vi "File HDF5 Close.vi"(8 "error in (no error)":errorcluster, 11 "HDF IDs in":T1) -> (0 "error out":errorcluster)   [LabVIEW 2011]
uses:
  Types Definitions/Type HDF IDs.ctl
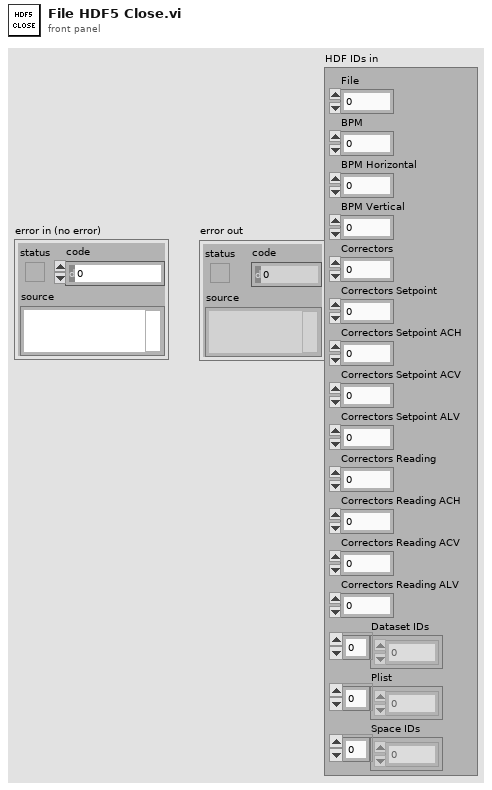
[diagram p1: front panel]
types:
  T1 = typedef "Type HDF IDs.ctl" = cluster{"File":i32, "BPM":i32, "BPM Horizontal":i32, "BPM Vertical":i32, "Correctors":i32, "Correctors Setpoint":i32, "Correctors Setpoint ACH":i32, "Correctors Setpoint ACV":i32, "Correctors Setpoint ALV":i32, "Correctors Reading":i32, "Correctors Reading ACH":i32, "Correctors Reading ACV":i32, "Correctors Reading ALV":i32, "Dataset IDs":i32[], "Plist":i32[], "Space IDs":i32[]}
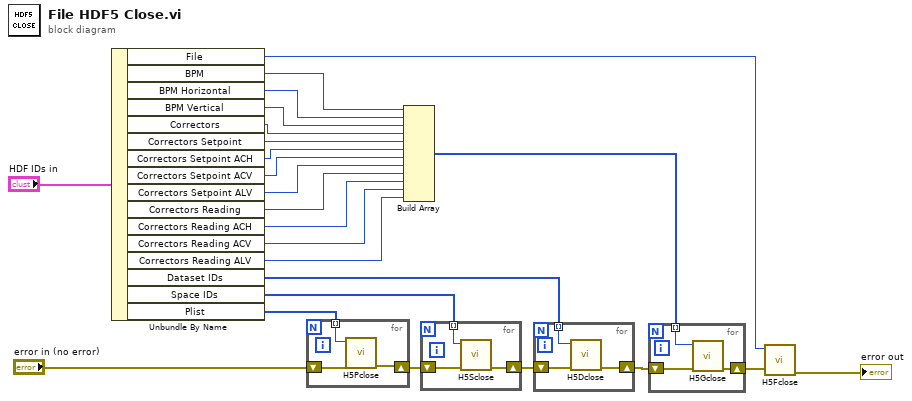
[diagram p0: block diagram]
diagram:
  n1 = Unbundle By Name("HDF IDs in") -> ("File"=w19:i32, "BPM"=w21:i32, "BPM Horizontal"=w20:i32, "BPM Vertical"=w18:i32, "Correctors"=w17:i32, "Correctors Setpoint"=w16:i32, "Correctors Setpoint ACH"=w15:i32, "Correctors Setpoint ACV"=w14:i32, "Correctors Setpoint ALV"=w13:i32, "Correctors Reading"=w12:i32, "Correctors Reading ACH"=w11:i32, "Correctors Reading ACV"=w10:i32, "Correctors Reading ALV"=w9:i32, "Dataset IDs"=w4:i32[], "Space IDs"=w3:i32[], "Plist"=w2:i32[])
  n2 = for {
    tunnel: w2 -> [w27] mode=indexing
    shift-right: [w25] -> w1
    shift-left: "error in (no error)" -> [w26]
    n3 = call <instrlib>:"H5Pclose.vi"("error in (no error)"=w26, "plist in"=w27) -> ("error out"=w25:errorcluster)  [unwired: 9 in]
  }
  n4 = Build Array(w21, w20, w18, w17, w16, w15, w14, w13, w12, w11, w10, w9) -> (w8:i32[])
  n5 = for {
    shift-right: [w28] -> w5
    shift-left: w1 -> [w29]
    tunnel: w3 -> [w30] mode=indexing
    n6 = call <instrlib>:"H5Sclose.vi"("error in (no error)"=w29, "space_id"=w30) -> ("error out"=w28:errorcluster)  [unwired: 9 in]
  }
  n7 = for {
    shift-right: [w33] -> w7
    shift-left: w5 -> [w32]
    tunnel: w4 -> [w31] mode=indexing
    n8 = call <instrlib>:"H5Dclose.vi"("error in (no error)"=w32, "dataset_id"=w31) -> ("error out"=w33:errorcluster)  [unwired: 9 in]
  }
  n9 = for {
    tunnel: w8 -> [w34] mode=indexing
    shift-right: [w36] -> w23
    shift-left: w7 -> [w35]
    n10 = call <instrlib>:"H5Gclose.vi"("error in (no error)"=w35, "group_id"=w34) -> ("error out"=w36:errorcluster)  [unwired: 9 in]
  }
  n11 = call <instrlib>:"H5Fclose.vi"("error in (no error)"=w23, "file_id"=w19) -> ("error out"=→"error out":errorcluster)  [unwired: 9 in]
